vi "家居.vi"() -> ()   [LabVIEW 2015]
uses:
  <vilib>/Instr/_visa.llb/VISA Configure Serial Port (Instr).vi
panel:
  out "湿度曲线":dbl[](graph)
  out "温度曲线":dbl[](graph)
  out "防盗":bool caption="量表"
  out "湿度/RH":dbl(knob) caption="量表" scale=0.0..100.0 scale format="%#.2g"
  in  "串口号：":refnum<visa-resource-name>
  out "温度/℃":dbl(knob) caption="量表" scale=0.0..50.0 scale format="%#.2g"
  # "基于Arduino与LabVIEW的智能家居系统"
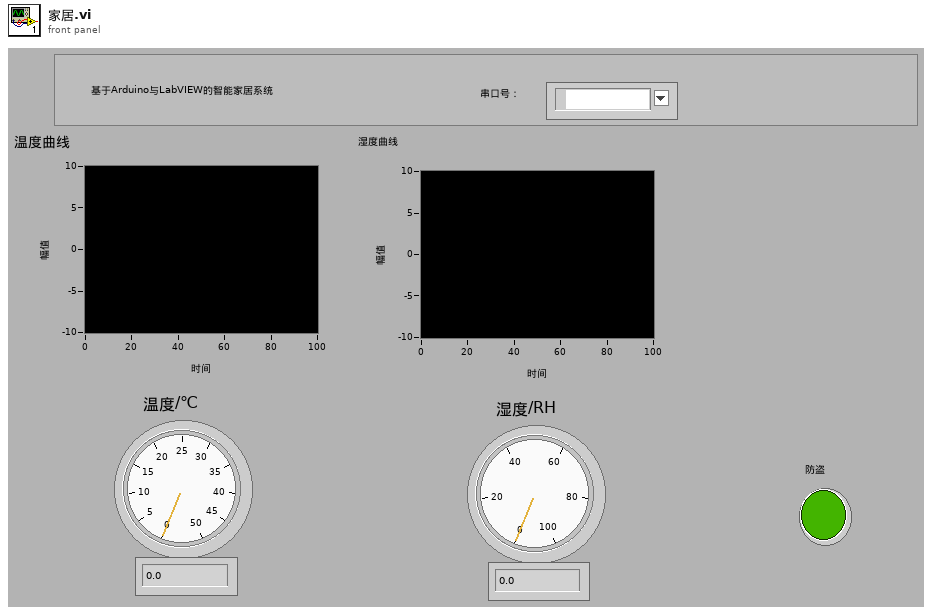
[diagram p1: front panel]
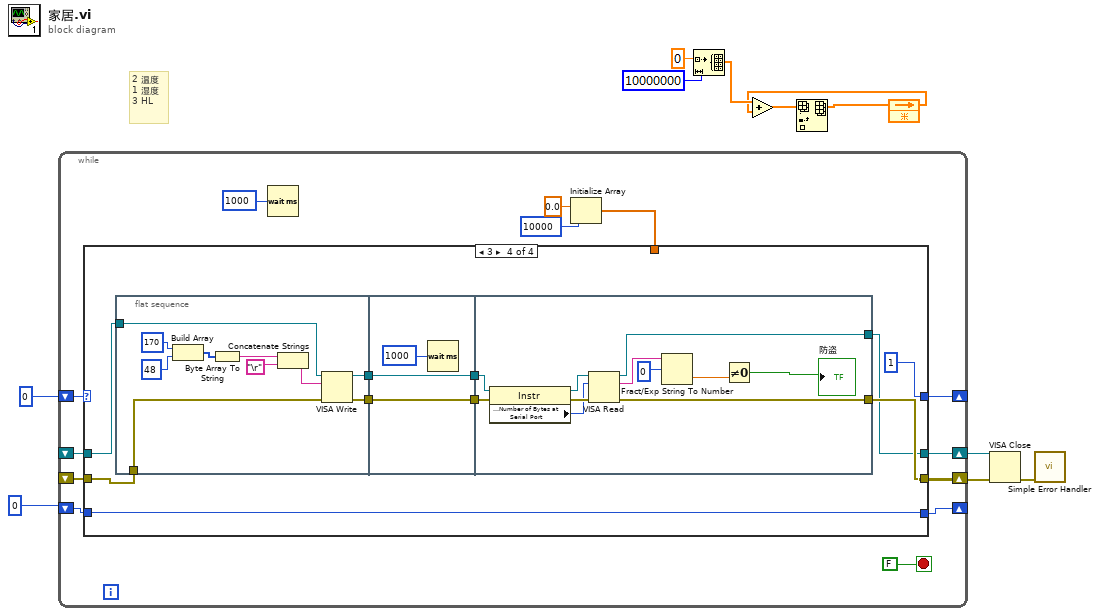
[diagram p0: block diagram]
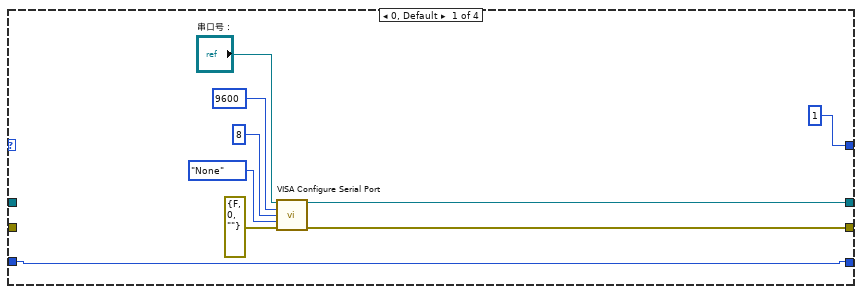
[diagram p2: hidden frame]
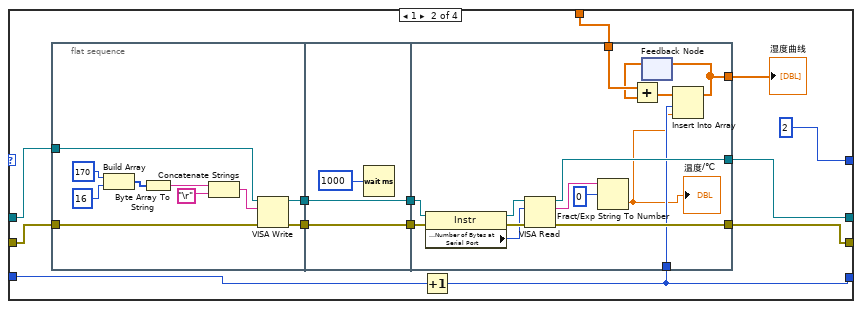
[diagram p3: hidden frame]
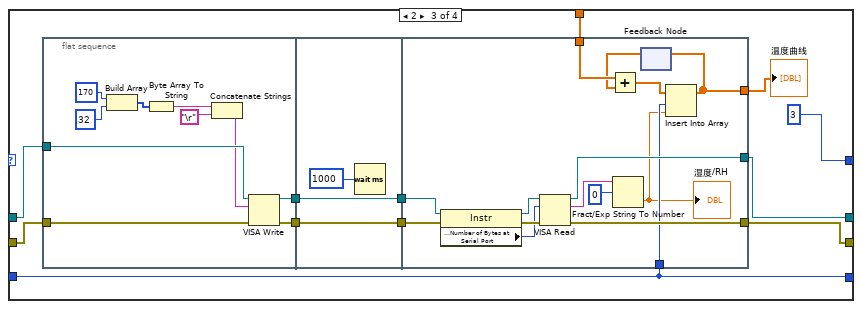
[diagram p4: hidden frame]
diagram:
  # "2 温度\n1 湿度\n3 HL"
  n1 = while {
    shift-right: [w18] -> w3
    shift-left: _ -> [w13]
    shift-right: [w17] -> w4
    shift-left: _ -> [w12]
    shift-right: [w16] -> _
    shift-left: 0 -> [w15]
    shift-right: [w6] -> _
    shift-left: 0 -> [w7]
    stop <- FALSE stop-if-true
    n2 = Wait (ms)(milliseconds to wait=u32 1000 ("等待时间（毫秒）")) -> ()  [unwired: 1 out]
    n3 = Initialize Array(0.0 ("元素"), 10000 ("维数大小")) -> (w10:dbl[])
    n4 = case shown="3" w15 {
      tunnel: [w23 w35 w75 w110] -> w18
      tunnel: [w22 w34 w74 w112] -> w17
      tunnel: [1 2 3 1] -> w16
      tunnel: w13 -> [_ w33 w73 w114]
      tunnel: w12 -> [_ w32 w72 w113]
      tunnel: w10 -> [_ w31 w71 _]
      tunnel: [w19 w28 w69 w109] -> w6
      tunnel: w7 -> [w19 w29 w69 w109]
      frame 0, Default {
        n5 = call-poly "VISA Configure Serial Port"("VISA resource name"="串口号：", "baud rate (9600)"=u32 9600, "data bits (8)"=u16 8, "parity (0:none)"=enum16{"None", "Odd", "Even", "Mark", "Space"}."None", "error in (no error)"=errorcluster {"status"=FALSE, "code"=0, "source"=""}) -> ("VISA resource name out"=w23:refnum<visa-resource-name>, "error out"=w22:errorcluster)  [unwired: 9 in]
      }
      frame 1 {
        n6 = flat-sequence {
          tunnel: w33 -> [w50]
          tunnel: w32 -> [w49]
          tunnel: [w48] -> w39
          tunnel: [w47] -> w38
          tunnel: w39 -> [w53]
          tunnel: w38 -> [w52]
          tunnel: [w53] -> w37
          tunnel: [w52] -> w36
          tunnel: w37 -> [w63]
          tunnel: w36 -> [w62]
          tunnel: [w61] -> w34
          tunnel: [w60] -> w35
          tunnel: w31 -> [w59]
          tunnel: [w56] -> w30
          tunnel: w28 -> [w55]
          frame #0 {
            n7 = Build Array(170, 16) -> (w45:i32[])
            n8 = Byte Array To String(unsigned byte array=w45) -> (string=w42:string)
            n9 = Concatenate Strings(w42, "\r") -> (w41:string)
            n10 = VISA Write(VISA resource name=w50, write buffer=w41, error in (no error)=w49) -> (VISA resource name out=w48:refnum<visa-resource-name>, error out=w47:errorcluster)  [unwired: 1 out]
          }
          frame #1 {
            n11 = Wait (ms)(milliseconds to wait=u32 1000 ("等待时间（毫秒）")) -> ()  [unwired: 1 out]
          }
          frame #2 {
            n12 = property class="Instr"(reference=w63, error in=w62) -> (reference out=w66:refnum<visa-resource-name>, error out=w65:errorcluster, "Serial Settings:Number of Bytes at Serial Port"=w64:u32)
            n13 = VISA Read(VISA resource name=w66, byte count=w64, error in (no error)=w65) -> (VISA resource name out=w60:refnum<visa-resource-name>, read buffer=w67:string, error out=w61:errorcluster)  [unwired: 1 out]
            n14 = Fract/Exp String To Number(string=w67, offset=0 ("偏移量")) -> (number=w54:dbl)  [unwired: 2 in, 1 out]
            "温度/℃" <- w54
            n15 = feedback #1() -> (w57:dbl[])  [unwired: 1 in]
            n16 = Add(x=w59, y=w57) -> (x+y=w58:dbl[])
            n17 = Insert Into Array(array=w58, index=w55, new element=w54) -> (w56:dbl[])
            n18 = feedback-in #1(w56) -> ()
          }
        }
        n19 = Increment(x=w29) -> (x+1=w28:i32)
        "湿度曲线" <- w30
      }
      frame 2 {
        n20 = flat-sequence {
          tunnel: w73 -> [w90]
          tunnel: w72 -> [w89]
          tunnel: [w88] -> w79
          tunnel: [w87] -> w78
          tunnel: w79 -> [w93]
          tunnel: w78 -> [w92]
          tunnel: [w93] -> w77
          tunnel: [w92] -> w76
          tunnel: w77 -> [w103]
          tunnel: w76 -> [w102]
          tunnel: [w101] -> w74
          tunnel: [w100] -> w75
          tunnel: w71 -> [w99]
          tunnel: w69 -> [w96]
          tunnel: [w94] -> w70
          frame #0 {
            n21 = Build Array(170, 32) -> (w85:i32[])
            n22 = Byte Array To String(unsigned byte array=w85) -> (string=w82:string)
            n23 = Concatenate Strings(w82, "\r") -> (w81:string)
            n24 = VISA Write(VISA resource name=w90, write buffer=w81, error in (no error)=w89) -> (VISA resource name out=w88:refnum<visa-resource-name>, error out=w87:errorcluster)  [unwired: 1 out]
          }
          frame #1 {
            n25 = Wait (ms)(milliseconds to wait=u32 1000 ("等待时间（毫秒）")) -> ()  [unwired: 1 out]
          }
          frame #2 {
            n26 = property class="Instr"(reference=w103, error in=w102) -> (reference out=w106:refnum<visa-resource-name>, error out=w105:errorcluster, "Serial Settings:Number of Bytes at Serial Port"=w104:u32)
            n27 = VISA Read(VISA resource name=w106, byte count=w104, error in (no error)=w105) -> (VISA resource name out=w100:refnum<visa-resource-name>, read buffer=w107:string, error out=w101:errorcluster)  [unwired: 1 out]
            n28 = Fract/Exp String To Number(string=w107, offset=0 ("偏移量")) -> (number=w95:dbl)  [unwired: 2 in, 1 out]
            "湿度/RH" <- w95
            n29 = feedback #2() -> (w97:dbl[])  [unwired: 1 in]
            n30 = Add(x=w99, y=w97) -> (x+y=w98:dbl[])
            n31 = Insert Into Array(array=w98, index=w96, new element=w95) -> (w94:dbl[])
            n32 = feedback-in #2(w94) -> ()
          }
        }
        "温度曲线" <- w70
      }
      frame 3 {
        (unwired) 1
        n33 = flat-sequence {
          tunnel: w114 -> [w128]
          tunnel: [w127] -> w118
          tunnel: [w126] -> w117
          tunnel: w113 -> [w125]
          tunnel: w118 -> [w131]
          tunnel: w117 -> [w130]
          tunnel: [w131] -> w116
          tunnel: [w130] -> w115
          tunnel: w116 -> [w137]
          tunnel: w115 -> [w136]
          tunnel: [w135] -> w112
          tunnel: [w134] -> w110
          frame #0 {
            n34 = Build Array(170, 48) -> (w123:i32[])
            n35 = Byte Array To String(unsigned byte array=w123) -> (string=w120:string)
            n36 = Concatenate Strings(w120, "\r") -> (w119:string)
            n37 = VISA Write(VISA resource name=w128, write buffer=w119, error in (no error)=w125) -> (VISA resource name out=w127:refnum<visa-resource-name>, error out=w126:errorcluster)  [unwired: 1 out]
          }
          frame #1 {
            n38 = Wait (ms)(milliseconds to wait=u32 1000 ("等待时间（毫秒）")) -> ()  [unwired: 1 out]
          }
          frame #2 {
            n39 = property class="Instr"(reference=w137, error in=w136) -> (reference out=w140:refnum<visa-resource-name>, error out=w139:errorcluster, "Serial Settings:Number of Bytes at Serial Port"=w138:u32)
            n40 = VISA Read(VISA resource name=w140, byte count=w138, error in (no error)=w139) -> (VISA resource name out=w134:refnum<visa-resource-name>, read buffer=w141:string, error out=w135:errorcluster)  [unwired: 1 out]
            n41 = Fract/Exp String To Number(string=w141, offset=0 ("偏移量")) -> (number=w133:dbl)  [unwired: 2 in, 1 out]
            n42 = Not Equal To 0?(x=w133) -> (x != 0?=→"防盗":bool)
          }
        }
      }
    }
  }
  n43 = VISA Close(VISA resource name=w3, error in (no error)=w4) -> (error out=w2:errorcluster)
  n44 = call <vilib>:"Simple Error Handler.vi"("error in (no error)"=w2) -> ()  [unwired: 4 in, 5 out]
